vi "Control Mode Write Array.vi"(8 "error in":errorcluster, 9 "Number of Channels":u32, 10 "Control Mode STS":u16, 11 "Power Supply In":refnum<class "Power Supply.lvclass">) -> (0 "error out":errorcluster, 3 "Power Supply Out":refnum<class "Power Supply.lvclass">)   [LabVIEW 2023, in "Power Supply.lvclass"]
uses:
  Power Supply.lvclass
  Power Supply.lvclass/Power Supply.ctl
  Low Level Capabilities/Control Mode/Control Mode.lvclass
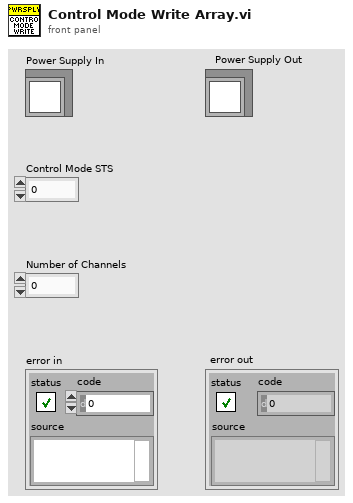
[diagram p1: front panel]
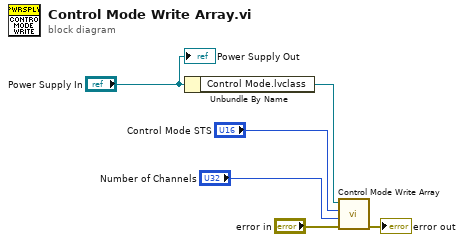
[diagram p0: block diagram]
diagram:
  n1 = Unbundle By Name("Power Supply In") -> ("Control Mode.lvclass"=w1:refnum<class "Control Mode.lvclass">)
  n2 = call-dynamic "Control Mode Write Array.vi"("error in"="error in", "Number of Channels"="Number of Channels", "Control Mode STS"="Control Mode STS", "Control Mode in"=w1) -> ("error out"=→"error out":errorcluster)  [unwired: 6 in, 1 out]
  "Power Supply Out" <- "Power Supply In"
